vi "Slack-files.upload.vi"(0 "token":string, 5 "channels":string, 7 "File":path, 11 "error in (no error)":errorcluster) -> (15 "error out":errorcluster)   [LabVIEW 2020]
uses:
  <vilib>/httpClient/MultipartData.ctl
  <vilib>/httpClient/LabVIEWHTTPClient.lvlib
panel:
  out "headers":string
  out "body":string
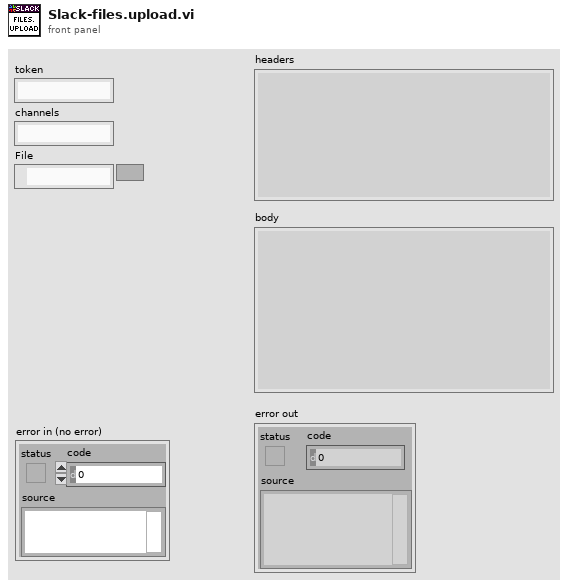
[diagram p1: front panel]
types:
  T1 = typedef "LabVIEWHTTPClient.lvlib/MultipartData.ctl" = cluster{"Name":string, "Value":string, "File":path, "Filename":string, "MIME type":string}
  T2 = typedef "LabVIEWHTTPClient.lvlib/ClientHandle.ctl" = refnum<k1>
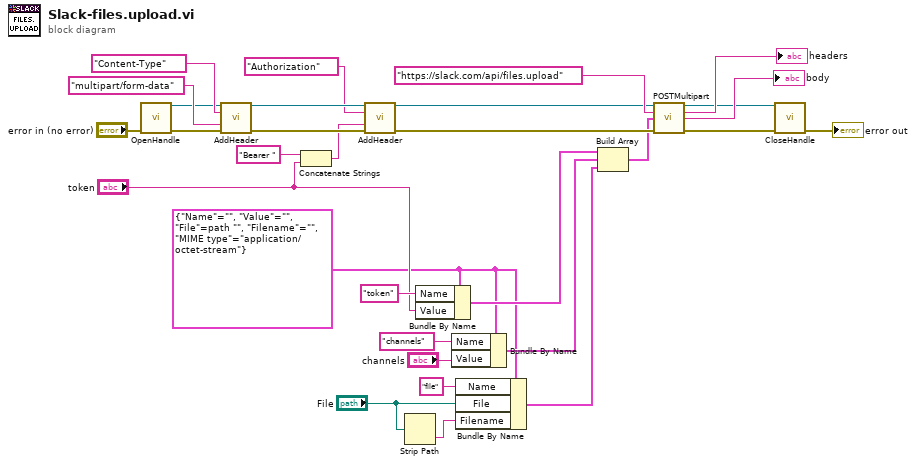
[diagram p0: block diagram]
diagram:
  w4 = T1 {"Name"="", "Value"="", "File"=path "", "Filename"="", "MIME type"="application/octet-stream"} ("Element")
  n1 = call <vilib>:"OpenHandle.vi"("error in (no error)"="error in (no error)") -> ("client handle out"=w25:T2, "error out"=w21:errorcluster)  [unwired: 13 in]
  n2 = call <vilib>:"AddHeader.vi"("client handle"=w25, "header"="Content-Type", "value"="multipart/form-data", "error in (no error)"=w21) -> ("client handle out"=w23:T2, "error out"=w22:errorcluster)  [unwired: 10 in]
  n3 = Concatenate Strings("Bearer " ("string"), "token") -> (w19:string)
  n4 = call <vilib>:"AddHeader.vi"("client handle"=w23, "header"="Authorization", "value"=w19, "error in (no error)"=w22) -> ("client handle out"=w24:T2, "error out"=w16:errorcluster)  [unwired: 10 in]
  n5 = Strip Path(path="File") -> (name=w10:string)  [unwired: 1 out]
  n6 = Bundle By Name(cluster=w4, "Name"="token", "Value"="token") -> (w13:T1)
  n7 = Bundle By Name(cluster=w4, "Name"="channels", "Value"="channels") -> (w5:T1)
  n8 = Bundle By Name(cluster=w4, "Name"="file", "File"="File", "Filename"=w10) -> (w3:T1)
  n9 = Build Array(w13, w5, w3) -> (w15:T1[])
  n10 = call <vilib>:"POSTMultipart.vi"("client handle"=w24, "url"="https://slack.com/api/files.upload", "data"=w15, "error in (no error)"=w16) -> ("client handle out"=w6:T2, "headers"=→"headers":string, "body"=→"body":string, "error out"=w8:errorcluster)  [unwired: 8 in]
  n11 = call <vilib>:"CloseHandle.vi"("client handle"=w6, "error in (no error)"=w8) -> ("error out"=→"error out":errorcluster)  [unwired: 13 in]
